vi "assemblies_features.vi"() -> ()   [LabVIEW 2019]
uses:
  <userlib>/IoT Devices/_subVIs/HTTPComm.ctl
  <userlib>/Onshape/_SubVI/Cluster.ctl
  <vilib>/Analysis/Matrix/Datatypes/RealMatrix.ctl
  <userlib>/Onshape/_SubVI/z did wid and eid.vi
  <vilib>/Analysis/Matrix/Numeric/Conversions/Array To Matrix - RA2.vi
  <vilib>/Analysis/Matrix/Numeric/Multiply/Multiply - RM,RM.vi
  <vilib>/Analysis/Matrix/NI_Matrix.lvlib
panel:
  out "Array 2":T1(array[cluster])
  out "A * B":T2
  out "init 2":dbl[][](array[numeric])
  out "init":dbl[][](array[numeric])
  out "element 2":T3
  out "element":T3
  out "Array":T4(array[cluster])
  out "Device  out":T5
  out "Comm":T6
  out "error out":errorcluster
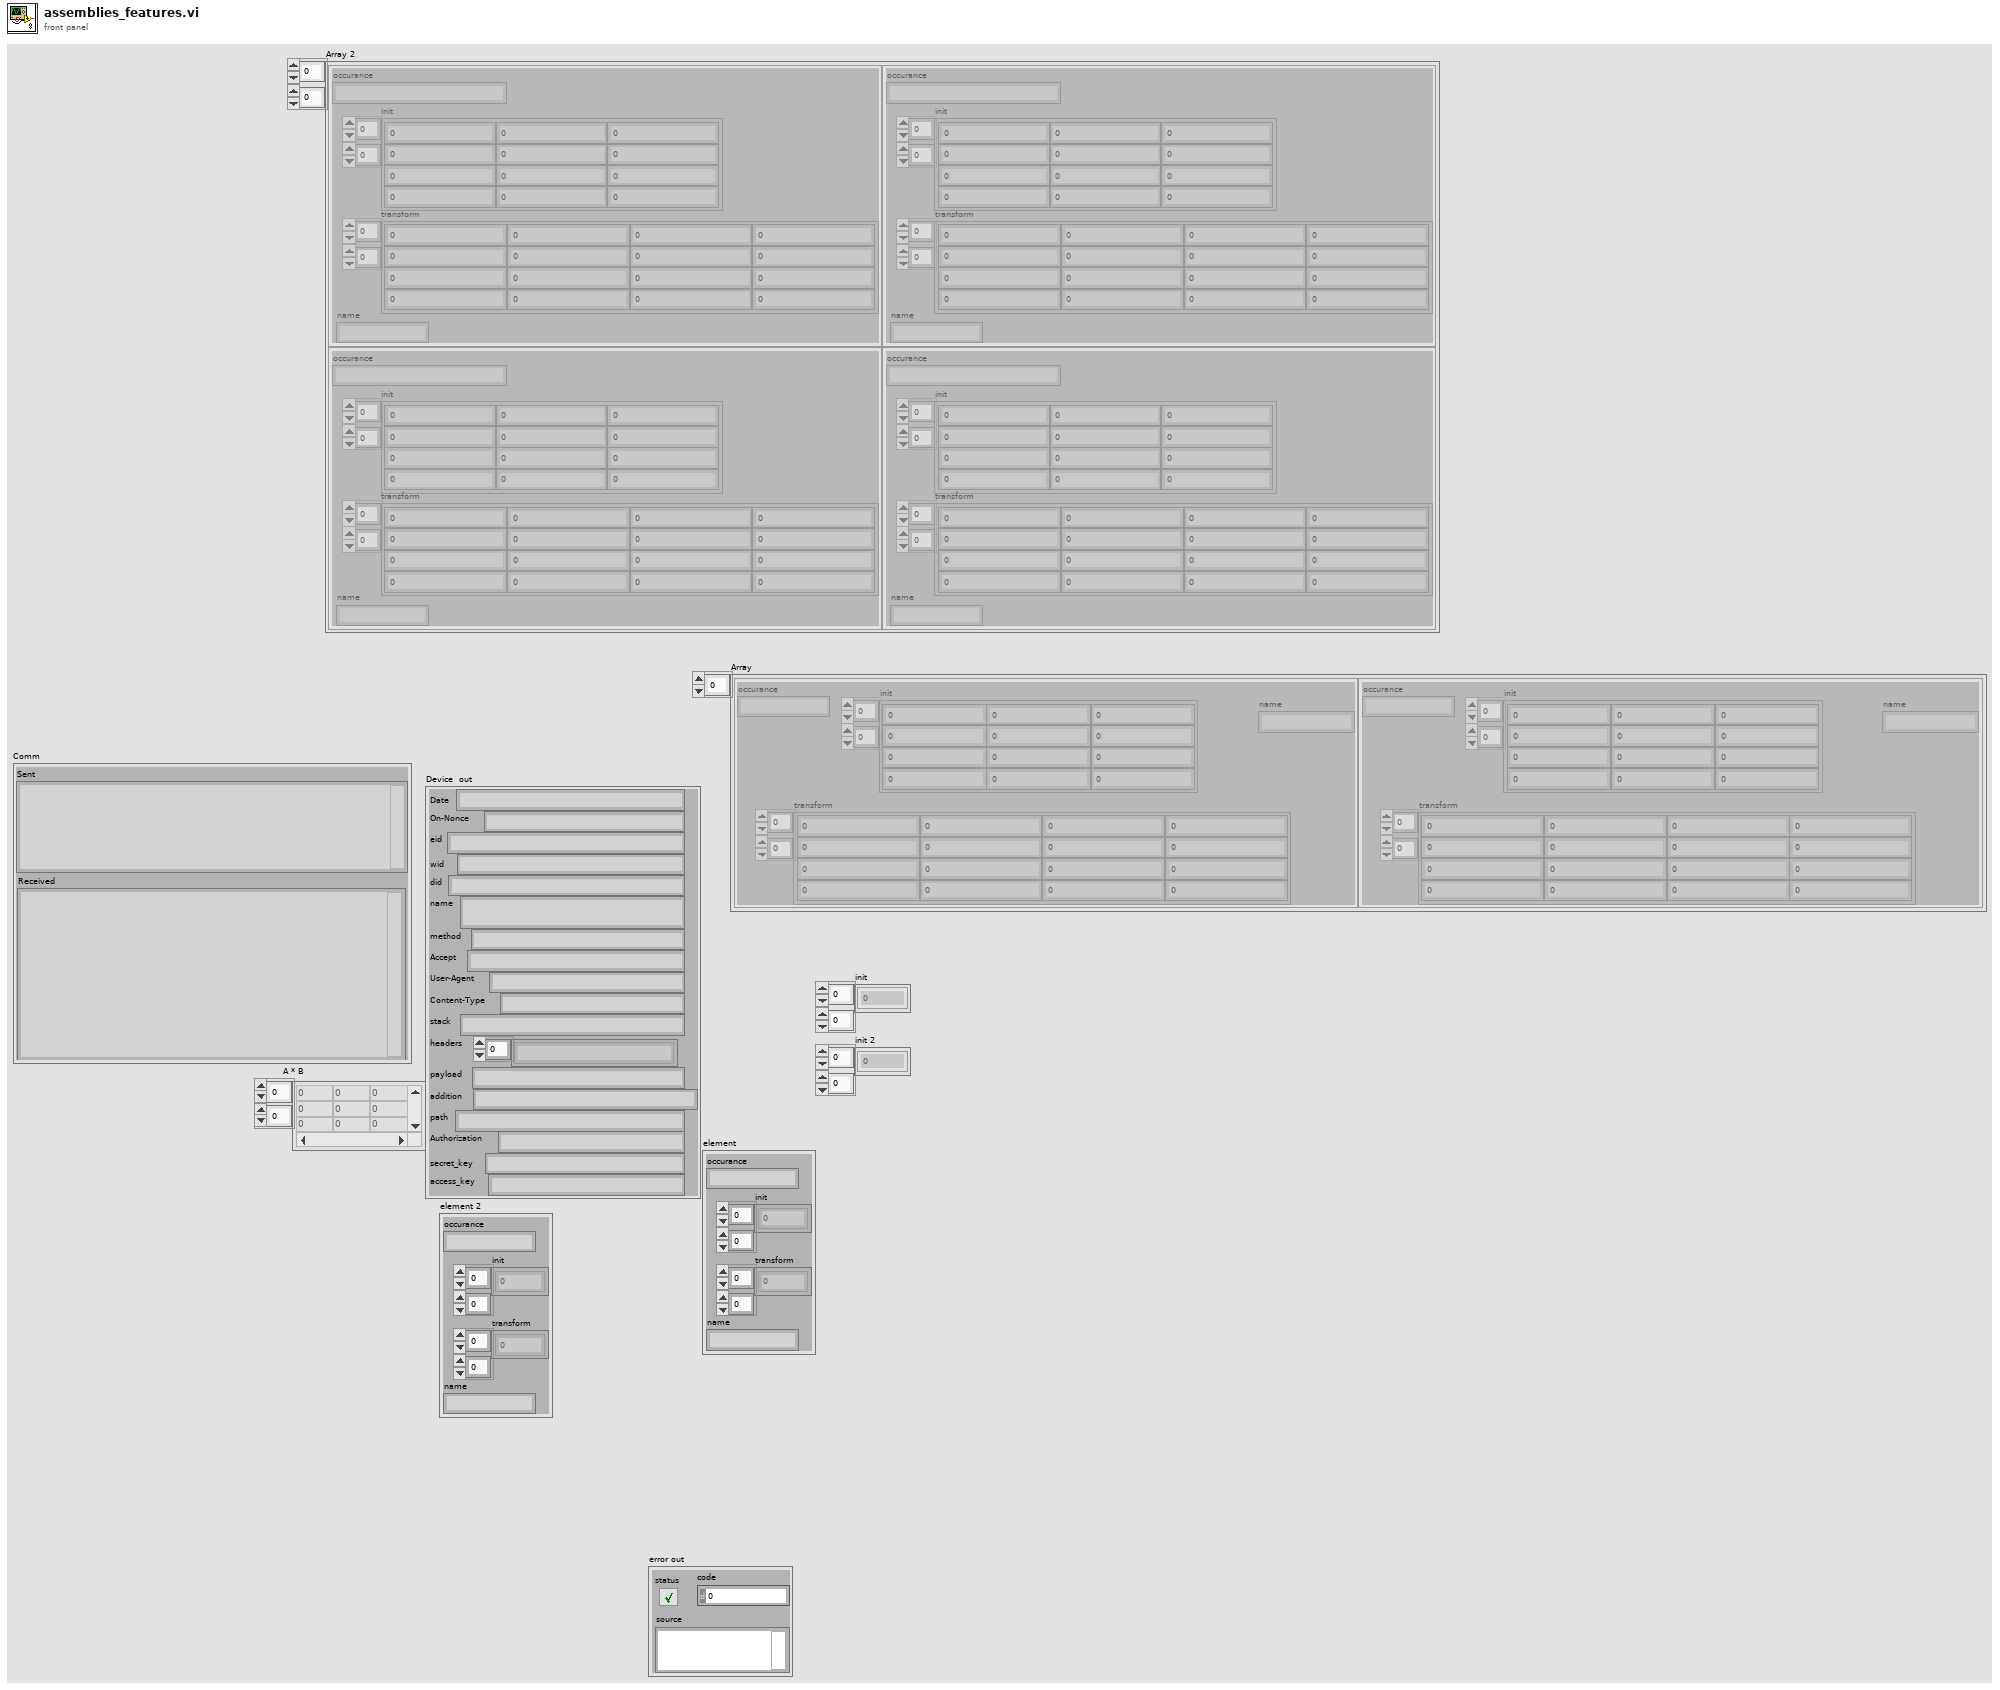
[diagram p1: front panel]
types:
  T1 = cluster{"occurance":string, "init":dbl[][], "transform":dbl[][], "name":string}[][]
  T2 = typedef "NI_Matrix.lvlib/RealMatrix.ctl" = dbl[][]
  T3 = cluster{"occurance":string, "init":dbl[][], "transform":dbl[][], "name":string}
  T4 = cluster{"occurance":string, "init":dbl[][], "transform":dbl[][], "name":string}[]
  T5 = typedef "Cluster.ctl" = cluster{"Date":string, "On-Nonce":string, "eid":string, "wid":string, "did":string, "name":string, "method":string, "Accept":string, "User-Agent":string, "Content-Type":string, "stack":string, "headers":string[], "payload":string, "addition":string, "path":string, "Authorization":string, "secret_key":string, "access_key":string}
  T6 = typedef "HTTPComm.ctl" = cluster{"url":string, "sent headers":string, "sent body":string, "headers":string, "body":string, "Sent":string, "Received":string}
  T7 = cluster{"rootAssembly":cluster{"elementId":string, "occurrences":cluster{"fixed":bool, "path":string[], "transform":dbl[]}[], "features":cluster{"featureData":cluster{"mateType":string, "matedEntities":cluster{"matedOccurrence":string[], "matedCS":cluster{"origin":dbl[], "xAxis":dbl[], "yAxis":dbl[], "zAxis":dbl[]}}[], "name":string}}[]}}
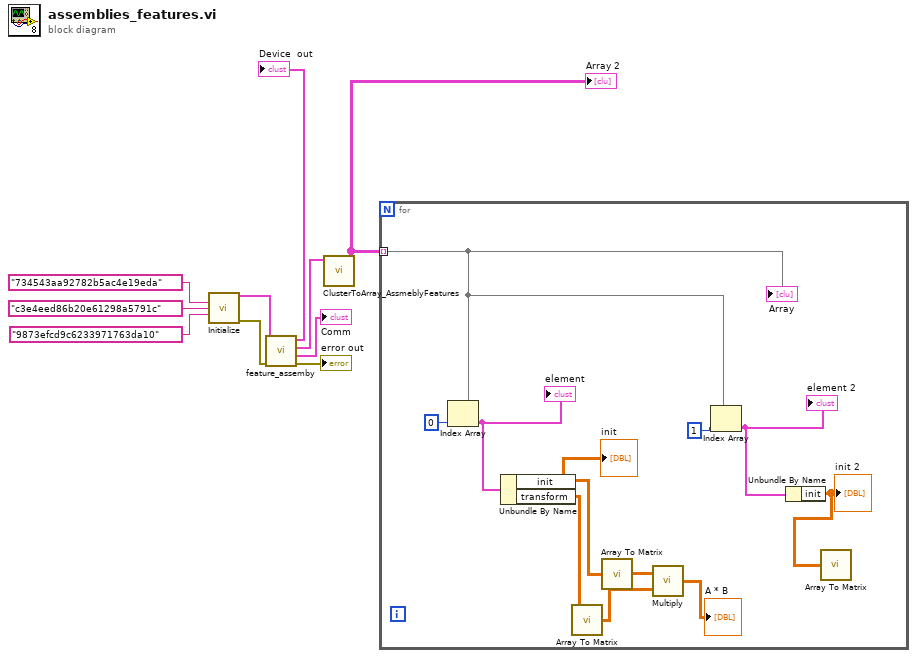
[diagram p0: block diagram]
diagram:
  n1 = call-poly <userlib>:"Initialize.vi"("did"="734543aa92782b5ac4e19eda", "wid"="c3e4eed86b20e61298a5791c", "eid"="9873efcd9c6233971763da10") -> ("Device Out"=w4:T5, "error out"=w3:errorcluster)  [unwired: 11 in]
  n2 = call <userlib>:"feature_assemby.vi"("error in (no error)"=w3, "Device Out in"=w4) -> ("error out"=→"error out":errorcluster, "Comm"=→"Comm":T6, "value"=w5:T7, "Device Out out"=→"Device  out":T5)  [unwired: 6 in]
  n3 = call <userlib>:"ClusterToArray_AssmeblyFeatures.vi"("value"=w5) -> ("Array"=w1:T1)  [unwired: 10 in]
  "Array 2" <- w1
  n4 = for {
    tunnel: w1 -> [w19] mode=indexing
    n5 = Index Array(array=w19, index=0) -> (element=w17:T3)
    "element" <- w17
    n6 = Unbundle By Name(w17) -> ("init"=w16:dbl[][], "transform"=w13:dbl[][])
    "init" <- w16
    n7 = call-poly <vilib>:"Array To Matrix.vi"("Real 2D Array"=w13) -> ("Real Matrix"=w12:T2)
    n8 = call-poly <vilib>:"Array To Matrix.vi"("Real 2D Array"=w16) -> ("Real Matrix"=w14:T2)
    n9 = call-poly <vilib>:"Multiply.vi"("Real Matrix B"=w12, "Real Matrix A"=w14) -> ("A * B"=→"A * B":T2)
    n10 = Index Array(array=w19, index=1) -> (element=w18:T3)
    "element 2" <- w18
    n11 = Unbundle By Name(w18) -> ("init"=w15:dbl[][])
    "init 2" <- w15
    n12 = call-poly <vilib>:"Array To Matrix.vi"("Real 2D Array"=w15) -> ()  [unwired: 1 out]
    "Array" <- w19
  }
